vi "FdxInitCvi.vi"(8 "error in":errorcluster) -> (0 "error out":errorcluster, 3 "Number of Servers":u32)   [LabVIEW 2020, in "AIM664LV.lvlib"]
doc: "This function initialises the entire application interface and must be called at first in an application program, before any other function is applied. This function returns the number of available servers."
uses:
  AIM664LV.lvlib
  FdxGlobalDllPath.vi
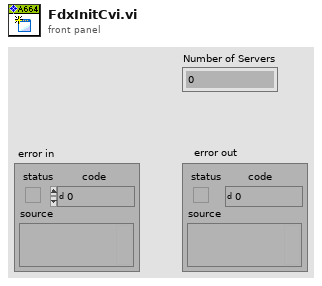
[diagram p1: front panel]
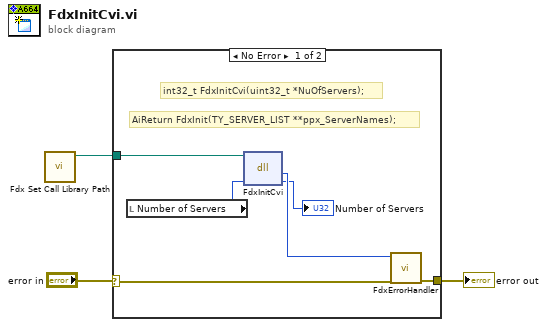
[diagram p0: block diagram]
diagram:
  n1 = call "Fdx Set Call Library Path.vi"() -> ("DllPath"=w1:path)  [unwired: 11 in]
  n2 = case shown="No Error" "error in" {
    selector: "error in" -> [w8 w10]
    tunnel: [w9 w10] -> w3
    tunnel: w1 -> [w4 _]
    frame No Error {
      # "AiReturn FdxInit(TY_SERVER_LIST **ppx_ServerNames);"
      # "int32_t FdxInitCvi(uint32_t *NuOfServers);"
      n3 = local read "Number of Servers"() -> (w5:u32)
      n4 = dll-call lib="aim_fdx.19.dll" fn="FdxInitCvi"(path in=w4, "NuOfServers"=w5) -> ("status"=w7:i32, "NuOfServers"=→"Number of Servers":u32)  [unwired: 2 in, 2 out]
      n5 = call "FdxErrorHandler.vi"("error in"=w8, "AIM Error"=w7) -> ("error out"=w9:errorcluster)  [unwired: 9 in]
    }
    frame Error {
    }
  }
  "error out" <- w3
